vi "SeleteUUT_DataSave.vi"(9 "选择测试板数据":dbl, 10 "测试步数":i32, 11 "real report 3":refnum<vi>) -> (1 "选择测试板数据 OUT":dbl, 2 "UUT OUT Data":string[][](array[string]), 3 "引用输出":refnum<vi>, 5 "PASS/FAIL":string)   [LabVIEW 2018]
panel:
  in  "real report":i32(listbox)
  out "元素":i32
  out "x*y":dbl
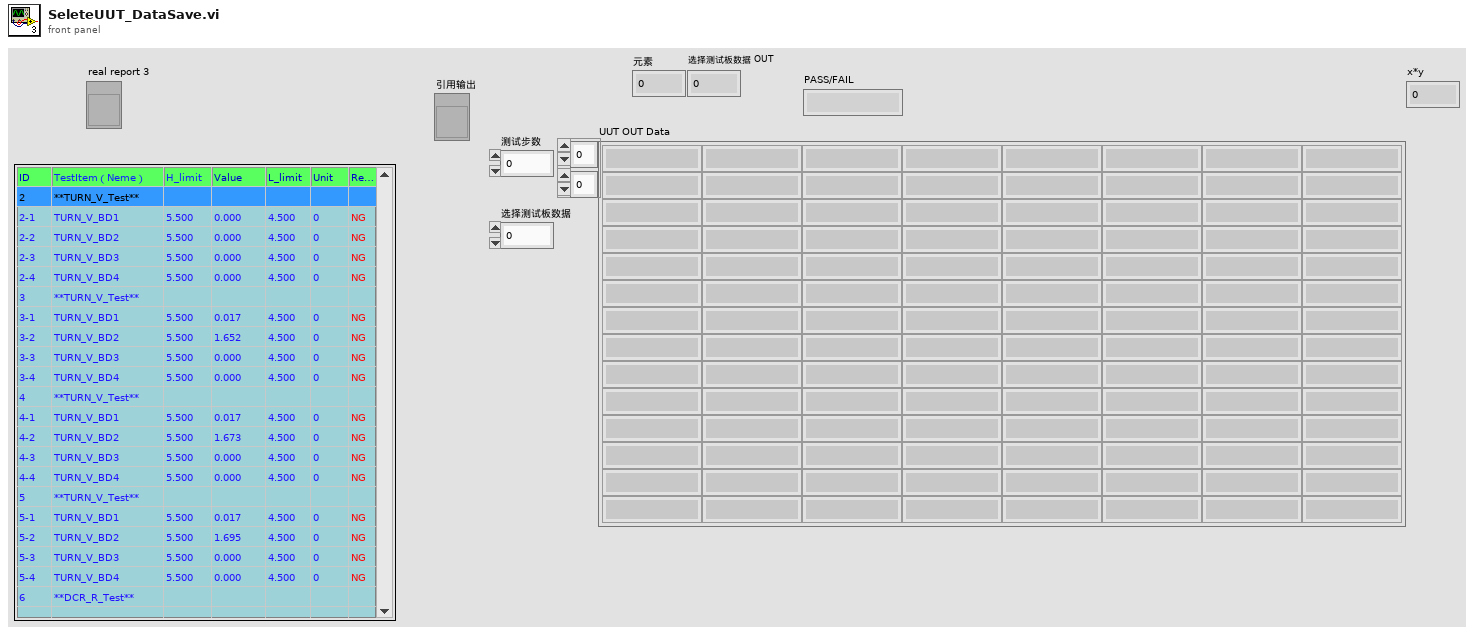
[diagram p1: front panel]
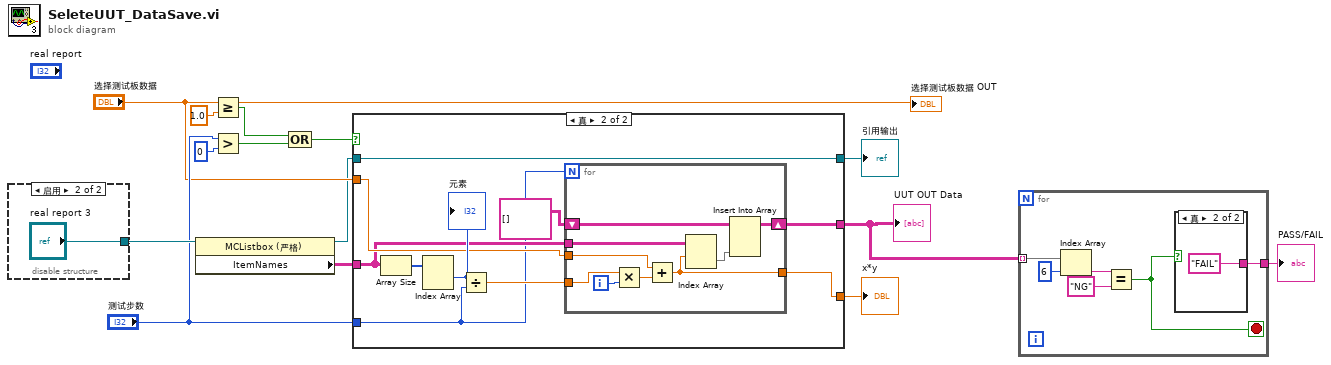
[diagram p0: block diagram]
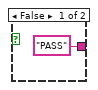
[diagram p2: hidden frame]
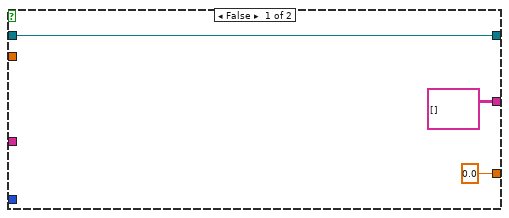
[diagram p3: hidden frame]
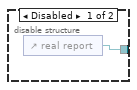
[diagram p4: hidden frame]
diagram:
  n1 = disable-structure shown="启用" {
    disable-tunnel: [w15 "real report 3"] -> w13
    frame Disabled {
      n2 = control-ref of="real report"() -> (w15:refnum<vi>)
    }
    frame Enabled {
    }
  }
  n3 = property class="MCListbox (严格)"(reference=w13) -> (reference out=w3:refnum<vi>, "ItemNames"=w12:string[][])  [unwired: 1 in, 1 out]
  n4 = Greater Or Equal?(x="选择测试板数据", y=1.0) -> (x >= y?=w5:bool)
  n5 = Greater?(x="测试步数", y=0) -> (0:w9:bool)
  n6 = Compound Arithmetic op=OR ("复合运算")(w5, w9) -> (w8:bool)
  n7 = case shown="真" w8 {
    tunnel: [string[][] [] ("项名") w26] -> w2
    tunnel: "测试步数" -> [_ w20]
    tunnel: "选择测试板数据" -> [_ w24]
    tunnel: [0.0 w23] -> w14
    tunnel: w12 -> [_ w22]
    tunnel: [w17 w21] -> w4
    tunnel: w3 -> [w17 w21]
    frame False {
    }
    frame True {
      n8 = Array Size(array=w22) -> (size(s)=w29:i32[])
      n9 = Index Array(array=w29) -> (element #1=w28:i32)  [unwired: 2 in, 1 out]
      "元素" <- w28
      n10 = Divide(x=w28, y=w20) -> (x/y=w25:dbl)
      n11 = for {
        N: w20 -> [_]
        tunnel: w22 -> [w38]
        tunnel: w25 -> [w37]
        shift-right: [w36] -> w26
        shift-left: string[][] [] ("项名") -> [w35]
        tunnel: w24 -> [w32]
        tunnel: [w30] -> w23
        i -> [w33]
        n12 = Multiply(x=w37, y=w33) -> (x*y=w31:dbl)
        n13 = Add(x=w32, y=w31) -> (x+y=w30:dbl)
        n14 = Index Array(array=w38, index (row)=w30) -> (element=w34:string[])  [unwired: 1 in]
        n15 = Insert Into Array(array=w35, new element=w34) -> (w36:string[][])  [unwired: 2 in]
      }
    }
  }
  "UUT OUT Data" <- w2
  "x*y" <- w14
  "引用输出" <- w4
  n16 = for {
    tunnel: w2 -> [w44] mode=indexing
    tunnel: [w39] -> w1
    stop <- w40 stop-if-true
    n17 = Index Array(array=w44, index=6 ("索引")) -> (element=w42:string)
    n18 = Equal?(x=w42, y="NG") -> (x = y?=w40:bool)
    n19 = case shown="真" w40 {
      tunnel: ["PASS" "FAIL"] -> w39
      frame False {
      }
      frame True {
      }
    }
  }
  "PASS/FAIL" <- w1
  "选择测试板数据 OUT" <- "选择测试板数据"
